vi "WPI_DMAResetStream.vi"(8 "error in (no error)":errorcluster, 11 "DMARef":T1) -> (0 "error out":errorcluster, 3 "DMARef":T1)   [LabVIEW 2017]
doc: "Removes all existing samples from the FPGA module on the roboRIO and the host buffer.\n\nThis software is licensed. Open the labview\\readme\\WPI Robotics Library Open Source License.txt file for more information."
uses:
  <vilib>/Rock Robotics/WPI/DMA/WPI_DMARef.ctl
  <vilib>/Rock Robotics/SystemInterfaces/DMA/FPGA_DMAWriteConfigOperation.ctl
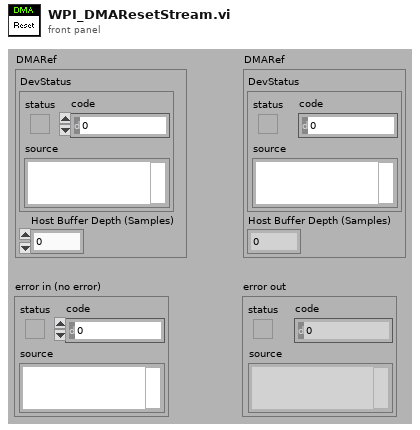
[diagram p1: front panel]
types:
  T1 = typedef "WPI_DMARef.ctl" = cluster{"DevStatus":errorcluster, "Host Buffer Depth (Samples)":u32}
  T2 = typedef "FPGA_DMAWriteConfigOperation.ctl" = enum16{"Update Pause", "Update Enable", "Update SampleClock"}
  T3 = typedef "FPGA_DMADevRef.ctl" = cluster{"DevStatus":errorcluster}
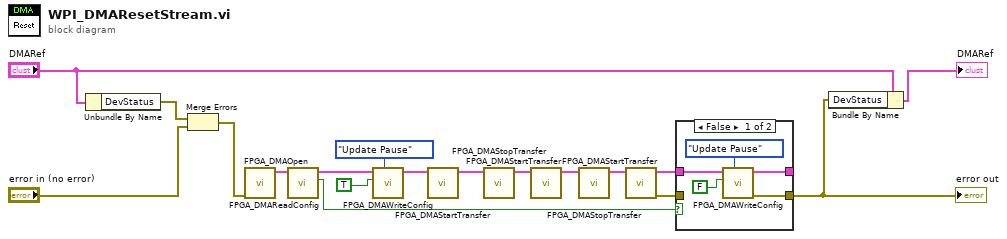
[diagram p0: block diagram]
diagram:
  n1 = Unbundle By Name("DMARef") -> ("DevStatus"=w3:errorcluster)
  n2 = Merge Errors(w3, "error in (no error)") -> (w2:errorcluster)
  n3 = call <vilib>:"FPGA_DMAOpen.vi"("error in (no error)"=w2) -> ("DMADevRef"=w7:T3)  [unwired: 10 out]
  n4 = call <vilib>:"FPGA_DMAReadConfig.vi"("DMADevRef In"=w7) -> ("Pause"=w5:bool, "DMADevRef Out"=w6:T3)  [unwired: 1 in, 8 out]
  n5 = call <vilib>:"FPGA_DMAWriteConfig.vi"("Operation"=FPGA_DMAWriteConfigOperation."Update Pause", "Pause"=TRUE, "DMADevRef"=w6) -> ("DMADevRef"=w9:T3)  [unwired: 3 in, 5 out]
  n6 = call <vilib>:"FPGA_DMAStartTransfer.vi"("DMADevRef In"=w9) -> ("DMADevRef Out"=w8:T3)  [unwired: 1 in, 9 out]
  n7 = call <vilib>:"FPGA_DMAStopTransfer.vi"("DMADevRef In"=w8) -> ("DMADevRef Out"=w13:T3)  [unwired: 1 in, 9 out]
  n8 = call <vilib>:"FPGA_DMAStartTransfer.vi"("DMADevRef In"=w13) -> ("DMADevRef Out"=w11:T3)  [unwired: 1 in, 9 out]
  n9 = call <vilib>:"FPGA_DMAStopTransfer.vi"("DMADevRef In"=w11) -> ("DMADevRef Out"=w12:T3)  [unwired: 1 in, 9 out]
  n10 = call <vilib>:"FPGA_DMAStartTransfer.vi"("DMADevRef In"=w12) -> ("error out"=w4:errorcluster, "DMADevRef Out"=w10:T3)  [unwired: 1 in, 8 out]
  n11 = case shown="False" w5 {
    tunnel: w10 -> [w21 w25]
    tunnel: [w20 w25] -> _
    tunnel: w4 -> [_ w24]
    tunnel: [w19 w24] -> w18
    frame False {
      n12 = call <vilib>:"FPGA_DMAWriteConfig.vi"("Operation"=FPGA_DMAWriteConfigOperation."Update Pause", "Pause"=FALSE, "DMADevRef"=w21) -> ("error out"=w19:errorcluster, "DMADevRef"=w20:T3)  [unwired: 3 in, 4 out]
    }
    frame True {
    }
  }
  "error out" <- w18
  n13 = Bundle By Name(cluster="DMARef", "DevStatus"=w18) -> (→"DMARef":T1)
